vi "ToyForStableDisplayOnGrabberAndSavingData.vi"() -> ()   [LabVIEW 2010]
panel:
  in  "Scanning":bool
  out "appended array":u32[](array[numeric])
  in  "s":bool
  out "Array 2":u32[](array[numeric])
  in  "stop":bool
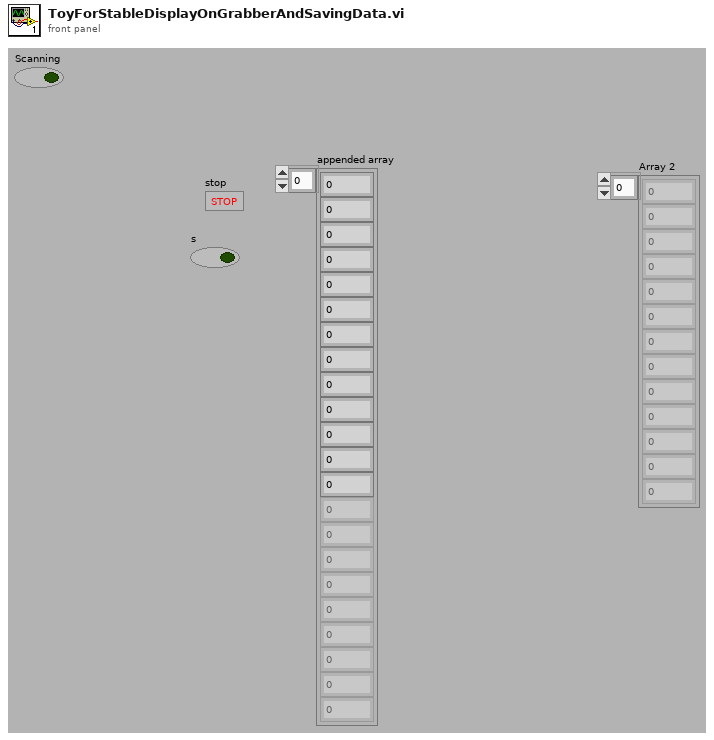
[diagram p1: front panel]
types:
  T1 = enum16{"open", "replace", "create", "open or create", "replace or create", "replace or create with confirmation"}
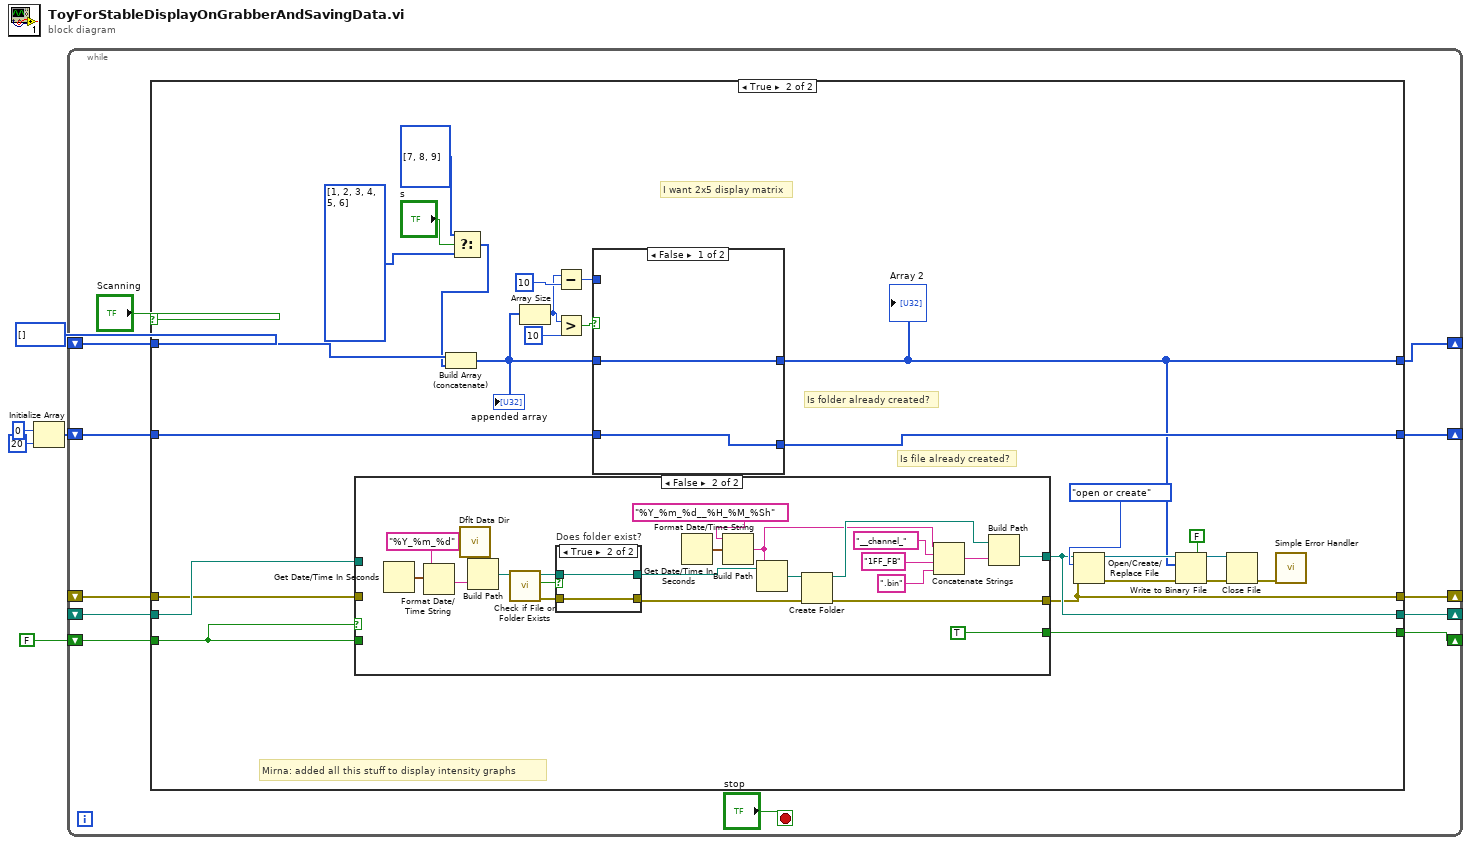
[diagram p0: block diagram]
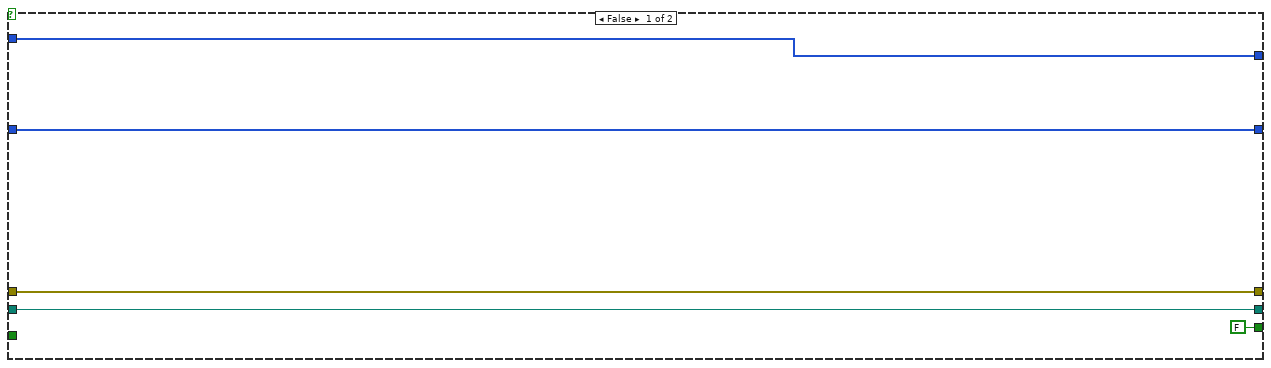
[diagram p2: hidden frame]
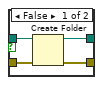
[diagram p4: hidden frame]
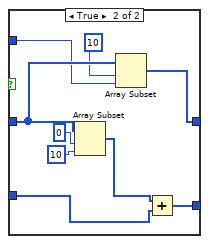
[diagram p5: hidden frame]
diagram:
  n1 = Initialize Array(u32 0 ("element"), 20 ("dimension size")) -> (w2:u32[])
  n2 = while {
    shift-right: [w15] -> _
    shift-left: u32[] [] -> [w16]
    shift-right: [w14] -> _
    shift-left: w2 -> [w13]
    shift-right: [w10] -> _
    shift-left: FALSE -> [w11]
    shift-right: [w9] -> _
    shift-left: _ -> [w8]
    shift-right: [w7] -> _
    shift-left: _ -> [w6]
    stop <- "stop" stop-if-true
    n3 = case shown="True" "Scanning" {
      tunnel: w16 -> [w22 w49]
      tunnel: [w22 w30] -> w15
      tunnel: [w21 w38] -> w14
      tunnel: w13 -> [w21 w37]
      tunnel: w11 -> [_ w27]
      tunnel: [FALSE ("FIFO overflow") w29] -> w10
      tunnel: [w19 w26] -> w9
      tunnel: w8 -> [w19 w25]
      tunnel: [w18 w24] -> w7
      tunnel: w6 -> [w18 w23]
      frame False {
      }
      frame True {
        # "Mirna: added all this stuff to display intensity graphs"
        # "Is folder already created?"
        # "Is file already created?"
        # "I want 2x5 display matrix"
        n4 = case shown="False" w27 {
          tunnel: [w50 w66] -> w24
          tunnel: w27 -> [w51 _]
          tunnel: [w51 TRUE ("FIFO overflow")] -> w29
          tunnel: [w52 w53] -> w26
          tunnel: w25 -> [w52 _]
          tunnel: w23 -> [w50 _]
          frame True {
          }
          frame False {
            n5 = Get Date/Time In Seconds() -> (seconds since 1Jan1904=w63:timestamp)
            n6 = Format Date/Time String(time format string (%c)="%Y_%m_%d", seconds (now)=w63) -> (date/time string=w64:string)  [unwired: 1 out]
            n7 = call <vilib>:"Dflt Data Dir.vi"() -> ("App:Default Data Directory"=w58:path)
            n8 = Build Path(base path=w58, name or relative path=w64) -> (appended path=w57:path)
            n9 = call <vilib>:"Check if File or Folder Exists.vi"("path"=w57) -> ("error out"=w59:errorcluster, "file or folder exists?"=w60:bool, "dup path"=w61:path)  [unwired: 1 in, 7 out]
            n10 = case "Does folder exist?" shown="True" w60 {
              tunnel: w59 -> [w78 w80]
              tunnel: w61 -> [w76 w79]
              tunnel: [w77 w80] -> w55
              tunnel: [w75 w79] -> w56
              frame False {
                n11 = Create Folder(path (use dialog)=w76, error in=w78) -> (created path=w75:path, error out=w77:errorcluster)  [unwired: 2 out]
              }
              frame True {
              }
            }
            n12 = Get Date/Time In Seconds() -> (seconds since 1Jan1904=w69:timestamp)
            n13 = Format Date/Time String(time format string (%c)="%Y_%m_%d__%H_%M_%Sh", seconds (now)=w69) -> (date/time string=w65:string)  [unwired: 1 out]
            n14 = Build Path(base path=w56, name or relative path=w65) -> (appended path=w68:path)
            n15 = Create Folder(path (use dialog)=w68, error in=w55) -> (created path=w67:path, error out=w66:errorcluster)  [unwired: 1 in, 1 out]
            n16 = Concatenate Strings(w65, "__channel_" ("string"), "1FF_FB" ("string"), ".bin" ("string")) -> (w71:string)
            n17 = Build Path(base path=w67, name or relative path=w71) -> (appended path=w53:path)
          }
        }
        n18 = Select(t=i32[] [7, 8, 9], s="s", f=i32[] [1, 2, 3, 4, 5, 6]) -> (s? t:f=w45:i32[])
        n19 = Build Array (concatenate)(w49, w45) -> (w44:u32[])
        "appended array" <- w44
        n20 = Array Size(array=w44) -> (size(s)=w40:i32)
        n21 = Subtract(x=w40, y=u8 10) -> (x-y=w39:i32)
        n22 = Greater?(x=w40, y=10) -> (0:w42:bool)
        n23 = case shown="False" w42 {
          tunnel: w44 -> [w82 w90]
          tunnel: [w82 w87] -> w30
          tunnel: w39 -> [_ w88]
          tunnel: [w81 w83] -> w38
          tunnel: w37 -> [w81 w85]
          frame False {
          }
          frame True {
            n24 = Array Subset(array=w90, index=0, length=10) -> (w84:u32[])
            n25 = Array Subset(array=w90, index=10, length=w88) -> (w87:u32[])
            n26 = Add(x=w84, y=w85) -> (x+y=w83:u32[])
          }
        }
        "Array 2" <- w30
        n27 = Open/Create/Replace File(file path (use dialog)=w26, error in=w24, operation (0:open)=T1."open or create") -> (refnum out=w31:refnum<file>, error out=w36:errorcluster)  [unwired: 3 in, 1 out]
        n28 = Write to Binary File(file (use dialog)=w31, data=w30, error in=w36, 5:FALSE ("prepend array or string size? (T)")) -> (refnum out=w32:refnum<file>, error out=w33:errorcluster)  [unwired: 2 in, 1 out]
        n29 = Close File(refnum=w32, error in=w33) -> (error out=w34:errorcluster)  [unwired: 1 out]
        n30 = call <vilib>:"Simple Error Handler.vi"("error in (no error)"=w34) -> ()  [unwired: 4 in, 5 out]
      }
    }
  }
